vi "Flow Sensors Control.vi"(5 "Initialized Array Cluster":T2, 7 "Initialized Index":i32, 11 "Slave Data Cluster":T1={"Current DoE"=[], "SSI 1 Flow Rate"=0.0, "SSI 2 Flow Rate"=0.0, "FLOM 1 Flow Rate"=0.0, "FLOM 2 Flow Rate"=0.0, "Pumps Running?"=FALSE, "Boolean 2"=FALSE, "Boolean 3"=FALSE, "Boolean 4"=FALSE, "At Equilibrium?"=FALSE, "Script Running?"=FALSE, "Current Script Iteration"=0.0, "Total Script Iterations"=0.0, "FLOM Pumps VISA"="COM2", "SSI 1 Pump VISA"="COM76", "SSI 2 Pump VISA"="COM74", "Huber Unistat VISA"="COM1", "SSI 3 Pump VISA"="COM76", "SSI 4 Pump VISA"="COM76", "SSI 4 Flow Rate"=0.0, "SSI 3 Flow Rate"=0.0, "Flow Meter 1 Rate "=0.0, "Flow Meter 2 Rate"=0.0, "Flow Meter 3 Rate"=0.0, "Flow Meter 4 Rate"=0.0, "SSI 1 Flow Setpoint"=0.0, "SSI 2 Flow Setpoint"=0.0, "SSI 3 Flow Setpoint"=0.0, "SSI 4 Flow Setpoint"=0.0, "Temperature Setpoint"=0.0, "Flow meter 1 COM"=15, "Flow meter 2 COM"=16, "Flow meter 4 COM"=19, "Flow meter 5 COM"=18, "Flow meter 3 COM"=17} {"Current DoE" format="%0.3f"}) -> (1 "Flow Rate Data Out":cluster{dbl, dbl, dbl, dbl, dbl}, 2 "Numeric out":i32, 3 "Flow Rate Data Array Cluster Out":T2)   [LabVIEW 2015]
uses:
  CFR LabVIEW Software/DoE_Control - JMW 03032016/DoE_Control_v5 Folder/DoE_Control - JMW 03092016/DoE_Control/000 Main Control - Mark Test/Standalone Control VI's/DoE_Control_Cluster.ctl
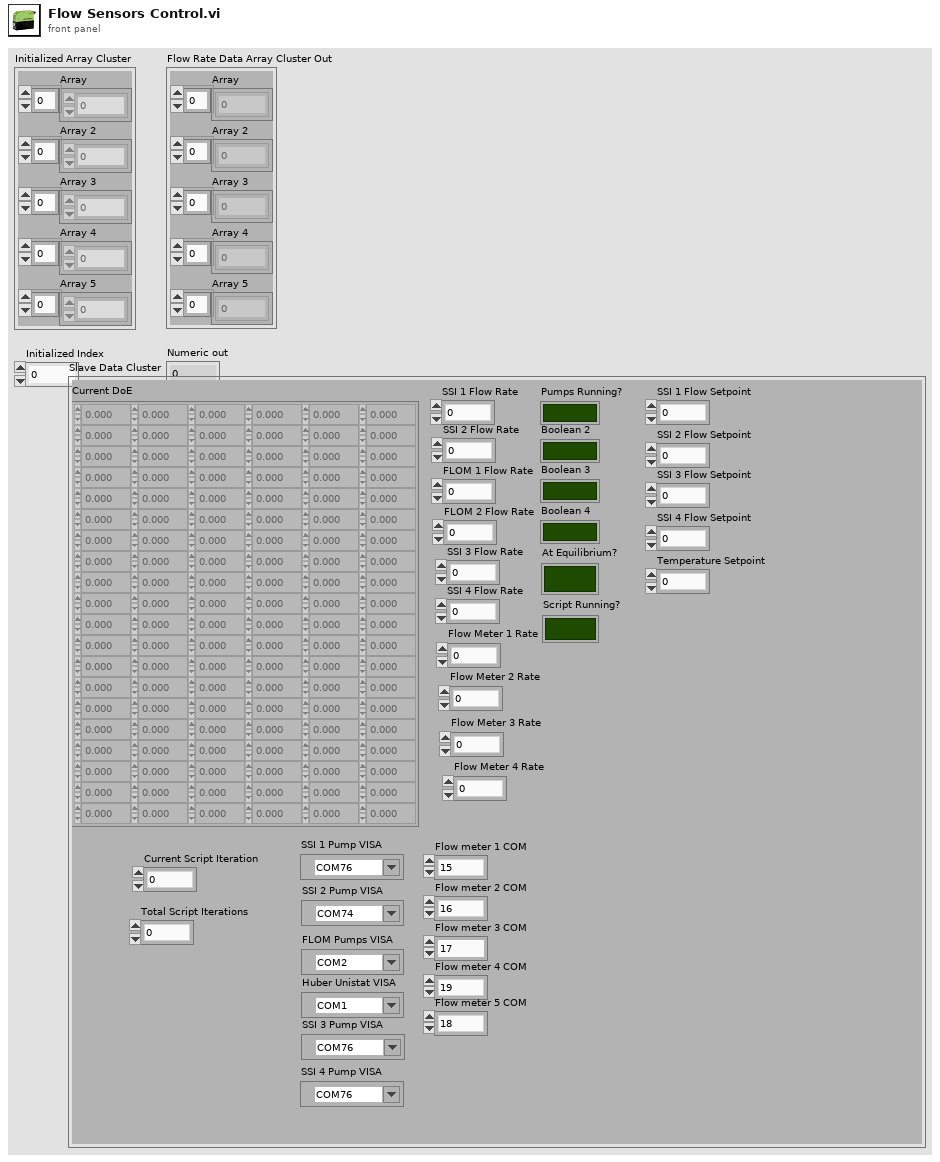
[diagram p1: front panel]
types:
  T1 = typedef "DoE_Control_Cluster.ctl" = cluster{"Current DoE":dbl[][], "SSI 1 Flow Rate":dbl, "SSI 2 Flow Rate":dbl, "FLOM 1 Flow Rate":dbl, "FLOM 2 Flow Rate":dbl, "Pumps Running?":bool, "Boolean 2":bool, "Boolean 3":bool, "Boolean 4":bool, "At Equilibrium?":bool, "Script Running?":bool, "Current Script Iteration":dbl, "Total Script Iterations":dbl, "FLOM Pumps VISA":refnum<visa-resource-name>, "SSI 1 Pump VISA":refnum<visa-resource-name>, "SSI 2 Pump VISA":refnum<visa-resource-name>, "Huber Unistat VISA":refnum<visa-resource-name>, "SSI 3 Pump VISA":refnum<visa-resource-name>, "SSI 4 Pump VISA":refnum<visa-resource-name>, "SSI 4 Flow Rate":dbl, "SSI 3 Flow Rate":dbl, "Flow Meter 1 Rate ":dbl, "Flow Meter 2 Rate":dbl, "Flow Meter 3 Rate":dbl, "Flow Meter 4 Rate":dbl, "SSI 1 Flow Setpoint":dbl, "SSI 2 Flow Setpoint":dbl, "SSI 3 Flow Setpoint":dbl, "SSI 4 Flow Setpoint":dbl, "Temperature Setpoint":dbl, "Flow meter 1 COM":u16, "Flow meter 2 COM":u16, "Flow meter 4 COM":u16, "Flow meter 5 COM":u16, "Flow meter 3 COM":u16}
  T2 = cluster{"Array":dbl[], "Array 2":dbl[], "Array 3":dbl[], "Array 4":dbl[], "Array 5":dbl[]}
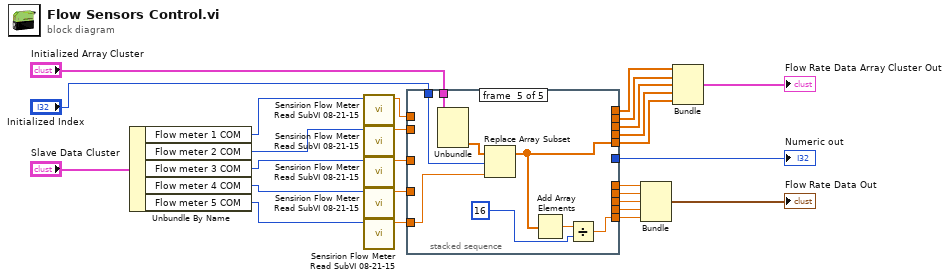
[diagram p0: block diagram]
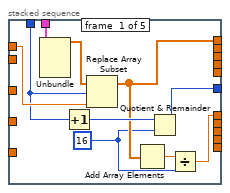
[diagram p2: hidden frame]
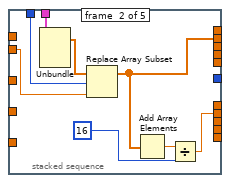
[diagram p3: hidden frame]
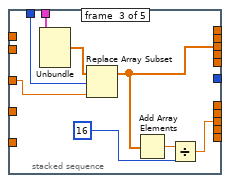
[diagram p4: hidden frame]
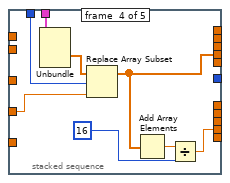
[diagram p5: hidden frame]
diagram:
  n1 = Unbundle By Name("Slave Data Cluster") -> ("Flow meter 1 COM"=w5:u16, "Flow meter 2 COM"=w4:u16, "Flow meter 3 COM"=w3:u16, "Flow meter 4 COM"=w2:u16, "Flow meter 5 COM"=w1:u16)
  n2 = call "Sensirion Flow Meter Read SubVI 08-21-15.vi"("COMPort"=w5) -> ("MeasureResult Scaled"=w8:dbl)  [unwired: 10 in]
  n3 = call "Sensirion Flow Meter Read SubVI 08-21-15.vi"("COMPort"=w4) -> ("MeasureResult Scaled"=w21:dbl)  [unwired: 10 in]
  n4 = call "Sensirion Flow Meter Read SubVI 08-21-15.vi"("COMPort"=w3) -> ("MeasureResult Scaled"=w22:dbl)  [unwired: 10 in]
  n5 = call "Sensirion Flow Meter Read SubVI 08-21-15.vi"("COMPort"=w2) -> ("MeasureResult Scaled"=w23:dbl)  [unwired: 10 in]
  n6 = call "Sensirion Flow Meter Read SubVI 08-21-15.vi"("COMPort"=w1) -> ("MeasureResult Scaled"=w24:dbl)  [unwired: 10 in]
  n7 = stacked-sequence {
    tunnel: [w32 _ _ _ _] -> w10
    tunnel: "Initialized Index" -> [w33 w44 w52 w60 w68]
    tunnel: [w35 _ _ _ _] -> w26
    tunnel: w8 -> [w34 _ _ _ _]
    tunnel: [w29 _ _ _ _] -> w9
    tunnel: "Initialized Array Cluster" -> [w28 w39 w49 w57 w65]
    tunnel: [_ w41 _ _ _] -> w11
    tunnel: [_ w40 _ _ _] -> w12
    tunnel: [_ _ w48 _ _] -> w15
    tunnel: [_ _ w47 _ _] -> w16
    tunnel: [_ _ _ w56 _] -> w17
    tunnel: [_ _ _ w55 _] -> w18
    tunnel: [_ _ _ _ w64] -> w19
    tunnel: [_ _ _ _ w62] -> w20
    tunnel: w21 -> [_ w37 _ _ _]
    tunnel: w22 -> [_ _ w45 _ _]
    tunnel: w23 -> [_ _ _ w53 _]
    tunnel: w24 -> [_ _ _ _ w61]
    frame #0 {
      w30 = 16 ("y")
      n8 = Unbundle(w28) -> ("Array"=w27:dbl[])  [unwired: 4 out]
      n9 = Increment(x=w33) -> (x+1=w36:i32)
      n10 = Replace Array Subset(array=w27, new element=w34, index=w33) -> (w32:dbl[])
      n11 = Add Array Elements(numeric array=w32) -> (sum=w31:dbl)
      n12 = Quotient & Remainder(x=w36, y=w30) -> (x-y*floor(x/y)=w35:i32)  [unwired: 1 out]
      n13 = Divide(x=w31, y=w30) -> (x/y=w29:dbl)
    }
    frame #1 {
      n14 = Unbundle(w39) -> ("Array 2"=w38:dbl[])  [unwired: 4 out]
      n15 = Replace Array Subset(array=w38, new element=w37, index=w44) -> (w40:dbl[])
      n16 = Add Array Elements(numeric array=w40) -> (sum=w43:dbl)
      n17 = Divide(x=w43, y=16) -> (x/y=w41:dbl)
    }
    frame #2 {
      n18 = Unbundle(w49) -> ("Array 3"=w46:dbl[])  [unwired: 4 out]
      n19 = Replace Array Subset(array=w46, new element=w45, index=w52) -> (w47:dbl[])
      n20 = Add Array Elements(numeric array=w47) -> (sum=w51:dbl)
      n21 = Divide(x=w51, y=16) -> (x/y=w48:dbl)
    }
    frame #3 {
      n22 = Unbundle(w57) -> ("Array 4"=w54:dbl[])  [unwired: 4 out]
      n23 = Replace Array Subset(array=w54, new element=w53, index=w60) -> (w56:dbl[])
      n24 = Add Array Elements(numeric array=w56) -> (sum=w59:dbl)
      n25 = Divide(x=w59, y=16) -> (x/y=w55:dbl)
    }
    frame #4 {
      n26 = Unbundle(w65) -> ("Array 5"=w63:dbl[])  [unwired: 4 out]
      n27 = Replace Array Subset(array=w63, new element=w61, index=w68) -> (w64:dbl[])
      n28 = Add Array Elements(numeric array=w64) -> (sum=w67:dbl)
      n29 = Divide(x=w67, y=16) -> (x/y=w62:dbl)
    }
  }
  "Numeric out" <- w26
  n30 = Bundle(w9, w11, w15, w18, w20) -> (→"Flow Rate Data Out":cluster{dbl, dbl, dbl, dbl, dbl})  [unwired: 1 in]
  n31 = Bundle("Array"=w10, "Array 2"=w12, "Array 3"=w16, "Array 4"=w17, "Array 5"=w19) -> (→"Flow Rate Data Array Cluster Out":T2)  [unwired: 1 in]
